vi "Configure IScan Trigger (Non-montonic Edge).vi"(0 "VISA resource name":refnum<visa-resource-name>, 5 "Channel (1: Channel1)":i32(ring)=1 items=["Channel1"=1, "Channel2"=2, "Channel3"=3, "Channel4"=4], 7 "Hysteresis Value (0 V)":dbl, 9 "Edge (0: Either)":i32(ring) items=["Either", "Falling", "Rising"], 11 "error in (no error)":errorcluster) -> (4 "VISA resource name out":refnum<visa-resource-name>, 15 "error out":errorcluster)   [LabVIEW 2013, in "Agilent 90000 Series.lvlib"]
doc: "Configures InfiniiScan trigger under non-montonic edge trigger mode."
uses:
  Agilent 90000 Series.lvlib
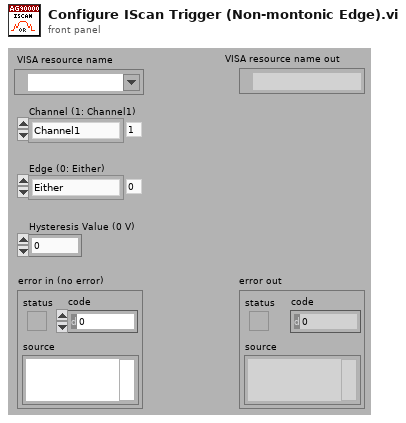
[diagram p1: front panel]
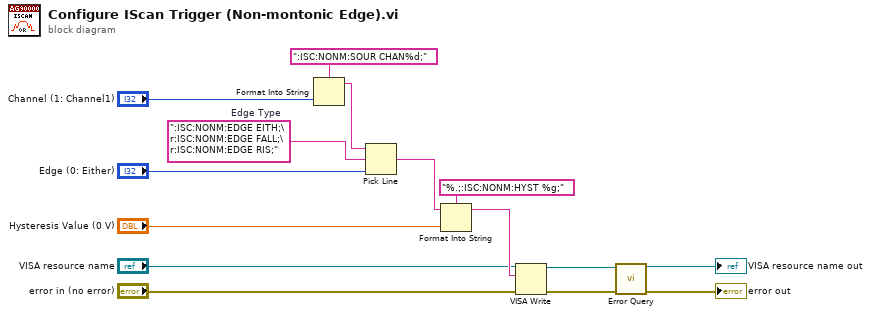
[diagram p0: block diagram]
diagram:
  w15 = ":ISC:NONM:EDGE EITH;\r:ISC:NONM:EDGE FALL;\r:ISC:NONM:EDGE RIS;"  # Edge Type
  n1 = Format Into String(format string=":ISC:NONM:SOUR CHAN%d;", "Channel (1: Channel1)") -> (resulting string=w1:string)  [unwired: 2 in, 1 out]
  n2 = Pick Line(string ("")=w1, multi-line string=w15, line index="Edge (0: Either)") -> (output string=w13:string)
  n3 = Format Into String(format string="%.;:ISC:NONM:HYST %g;", initial string=w13, "Hysteresis Value (0 V)") -> (resulting string=w10:string)  [unwired: 1 in, 1 out]
  n4 = VISA Write(VISA resource name="VISA resource name", write buffer=w10, error in (no error)="error in (no error)") -> (VISA resource name out=w7:refnum<visa-resource-name>, error out=w6:errorcluster)  [unwired: 1 out]
  n5 = call "Error Query.vi"("error in (no error)"=w6, "VISA resource name"=w7) -> ("error out"=→"error out":errorcluster, "VISA resource name out"=→"VISA resource name out":refnum<visa-resource-name>)  [unwired: 8 out]
